vi "PH_Beamline.color PA BL.vi"(0 "i ref in":refnum<vi>, 2 "Color State PA Input":i32, 5 "error in (no error)":errorcluster) -> (14 "i ref out":refnum<vi>, 16 "Color State PA Exit to ED":i32, 17 "Color State PA Exit to MA":i32, 18 "Color State PA Exit to Lab":i32, 19 "error out":errorcluster)   [LabVIEW 2014, in "PH_Beamline.lvlib"]
doc: "This Vi colors the PreAmp beamline elements."
uses:
  PH_Beamline.lvlib
  PH_StatusHandler/PH_StatusHandler.Status.ctl
  PH_Common/PH_Common.lvlib
  PH_BL-Master/PH_BL-Master.lvlib
  PH_StatusHandler/PH_StatusHandler.lvlib
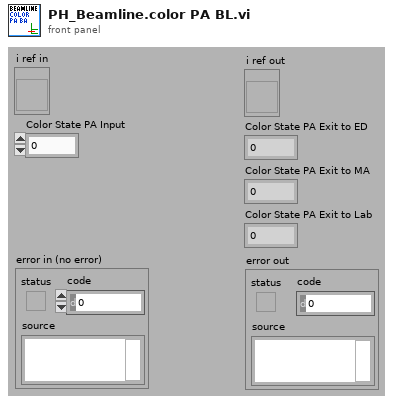
[diagram p1: front panel]
types:
  T1 = typedef "PH_StatusHandler.lvlib/PH_StatusHandler.Status.ctl" = i16
  T2 = typedef "PH_Beamline.lvlib/PH_Beamline.i attribute.ctl" = cluster{"GUI Refs":cluster{"PA ok":refnum<vi>, "MA ok":refnum<vi>, "fs FE ok":refnum<vi>, "ns FE ok":refnum<vi>, "PA ED ok":refnum<vi>, "MAS ok":refnum<vi>, "Booster ok":refnum<vi>, "Mirrortower ok":refnum<vi>, "In.-Box ok":refnum<vi>, "Compressor ok":refnum<vi>, "Experiment LB ok":refnum<vi>, "Experiment LL ok":refnum<vi>, "PHELIX_Beckhoff_Watchdog":refnum<vi>, "Shutters closed":refnum<vi>, "uOPA ok":refnum<vi>, "Vacuum no shotcond Comp LB":refnum<vi>}, "Refs BL MA":refnum<vi>[], "Refs BL MA-IB":refnum<vi>[], "Refs BL fs":refnum<vi>[], "Refs BL PA ED":refnum<vi>[], "Refs BL MAS":refnum<vi>[], "Refs BL Boo":refnum<vi>[], "Refs BL ns":refnum<vi>[], "Refs BL Mirrortower":refnum<vi>[], "Refs BL Compressor":refnum<vi>[], "Refs BL Exp LB":refnum<vi>[], "Radiation Safety":cluster{"Exp Laserbay":cluster{"Ref Op Mode":refnum<vi>, "Ref Laserbay evacuated":refnum<vi>, "Tagname LB evacuated":string, "Shot Mode":T3, "Laserbay evacuated?":i32, "Tagname HV room locked":string, "HV room locked?":i32, "Ref HV room locked":refnum<vi>, "Tagname bridged?":string, "Ref Bridge":refnum<vi>, "I<1E18W/cm²":bool}, "Exp Laserlab":cluster{"Ref Op Mode":refnum<vi>, "Ref Laserlab evacuated":refnum<vi>, "Tagname LL evacuated":string, "Shot Mode":T3, "Laserlab evacuated?":i32, "Tagname bridged?":string, "Ref Bridge":refnum<vi>, "I<1E18W/cm²":bool}}, "Refs BL LL":refnum<vi>[], "PP Igni Heating GUI Refs":refnum<vi>[], "PP Igni Heating Tagnames ":string[], "Refs BL PA":cluster{"undelayed Line before Shutter":refnum<vi>[], "undelayed Line after Shutter":refnum<vi>[], "before Bypass":refnum<vi>[], "delayed Line before Shutter":refnum<vi>[], "delayed Line after Shutter":refnum<vi>[], "before Shutter Input":refnum<vi>[], "after Shutter Input":refnum<vi>[], "Bypass":refnum<vi>[], "before Shutter Exit":refnum<vi>[], "after Shutter Exit":refnum<vi>[], "to MA":refnum<vi>[], "to Lab":refnum<vi>[]}, "BL":cluster{"YLF_BL_Status":i32, "fs_BL_Status":i32, "fs_YLF_BL_Status":i32, "ns_BL_Status":i32, "PA_Input_BL_Status":i32, "PA_UnDelay_BL_Status":i32, "PA_Delay_BL_Status":i32, "PA_BL_Status":i32, "PA_Bypass_BL_Status":i32, "PA_Exit_BL_Status":i32, "PA_LL_BL_Status":i32, "LL_BL_Status":i32, "PA_MA_BL_Status":i32, "MA_Exit_BL_Status":i32, "MA_Z6_BL_Status":i32, "Z6_BL_Status":i32, "MA_LB_BL_Status":i32, "LB_TB2_BL_Status":i32, "PA_before_Bypass_BL_Status":i32, "LB_TB3_BL_Status":i32}, "State Subsystems":cluster{"PA":bool, "MA":bool, "ns FE":bool, "fs FE":bool, "PA ED":bool, "In.-Box":bool, "MAS":bool, "Booster":bool, "Mirrortower":bool, "Compressor":bool, "Experiment LB":bool, "Experiment LL":bool, "uOPA":bool}, "Status Subscriber Information":T4, "Refs BL uOPA":refnum<vi>[], "PA_Input_2_Beam_6PWpGUI not linked?":bool, "PA_Input_Delay_6PGUI not linked?":bool, "Settings":T7}
  T3 = typedef "PH_Beamline.lvlib/PH_Beamline.Operation Mode.ctl" = i32
  T4 = typedef "PH_Beamline.lvlib/PH_Beamline.Status Subscriber Information.ctl" = cluster{"fs Swich YLF":T5, "fs Exit Shutter":T5, "ns Exit Shutter":T5, "PA Input Shutter":T5, "PA PC WP":T5, "PA PC WP 2":T5, "PA Bypass In":T5, "PA Bypass Out":T5, "PA CH 1":T5, "PA delayed":T5, "PA non delayed":T5, "PA Exit Shutter":T5, "PA Switch Lab":T5, "PA Bridge CH Input MA":T5, "MA Diffusor IB":T5, "MA IB Ready":T5, "MA CH 1":T5, "MA CH 2":T5, "MA CH 3":T5, "MA CH 4":T5, "MA Shutter Align Cam":T5, "MA Position MM5":T5, "Calorimeter Switch":T5, "BL Z6 CH 9":T5, "BL Z6 Beamdump":T5, "BL Z6 Shutter":T5, "COS Sensitivity Switch":T5, "Exp LB Shutter":T5, "Exp LB TB 2":T5, "Exp LB TB 3":T5, "PA LL Input CH":T5, "PA LL Output CH":T5, "LL Comp Input Shutter":T5, "LL Comp Output Shutter":T5, "LL Comp FF Shutter":T5, "Exp LL Shutter":T5, "MA IM In IB":T5, "MA IM Out IB":T5, "MA DB In IB":T5, "MA DB Out IB":T5, "Exp LB Shutter Interlock":T5, "Exp LL Shutter Interlock":T5, "MM1 Force Sensor":T5}
  T5 = typedef "PH_BL-Master.lvlib/PH_BL-Master.Status Subscriber Information.ctl" = cluster{"Index of element":i32, "Attributeset":T6}
  T6 = typedef "PH_BL-Master.lvlib/PH_BL-Master.Attribute Set.ctl" = enum16{"Boolean Status Service Subscriber", "Picture Status Service Subscriber"}
  T7 = typedef "PH_Beamline_Chief.lvlib/PH_Beamline_Chief.Settings.ctl" = cluster{"PA Doublepass Mode":bool, "Compressor Vaccuum LB not relevant":bool, "Windowshutter TB2 not relevant":bool, "Windowshutter TB3 not relevant":bool}
  T8 = cluster{"YLF_BL_Status":i32, "fs_BL_Status":i32, "fs_YLF_BL_Status":i32, "ns_BL_Status":i32, "PA_Input_BL_Status":i32, "PA_UnDelay_BL_Status":i32, "PA_Delay_BL_Status":i32, "PA_BL_Status":i32, "PA_Bypass_BL_Status":i32, "PA_Exit_BL_Status":i32, "PA_LL_BL_Status":i32, "LL_BL_Status":i32, "PA_MA_BL_Status":i32, "MA_Exit_BL_Status":i32, "MA_Z6_BL_Status":i32, "Z6_BL_Status":i32, "MA_LB_BL_Status":i32, "LB_TB2_BL_Status":i32, "PA_before_Bypass_BL_Status":i32, "LB_TB3_BL_Status":i32}
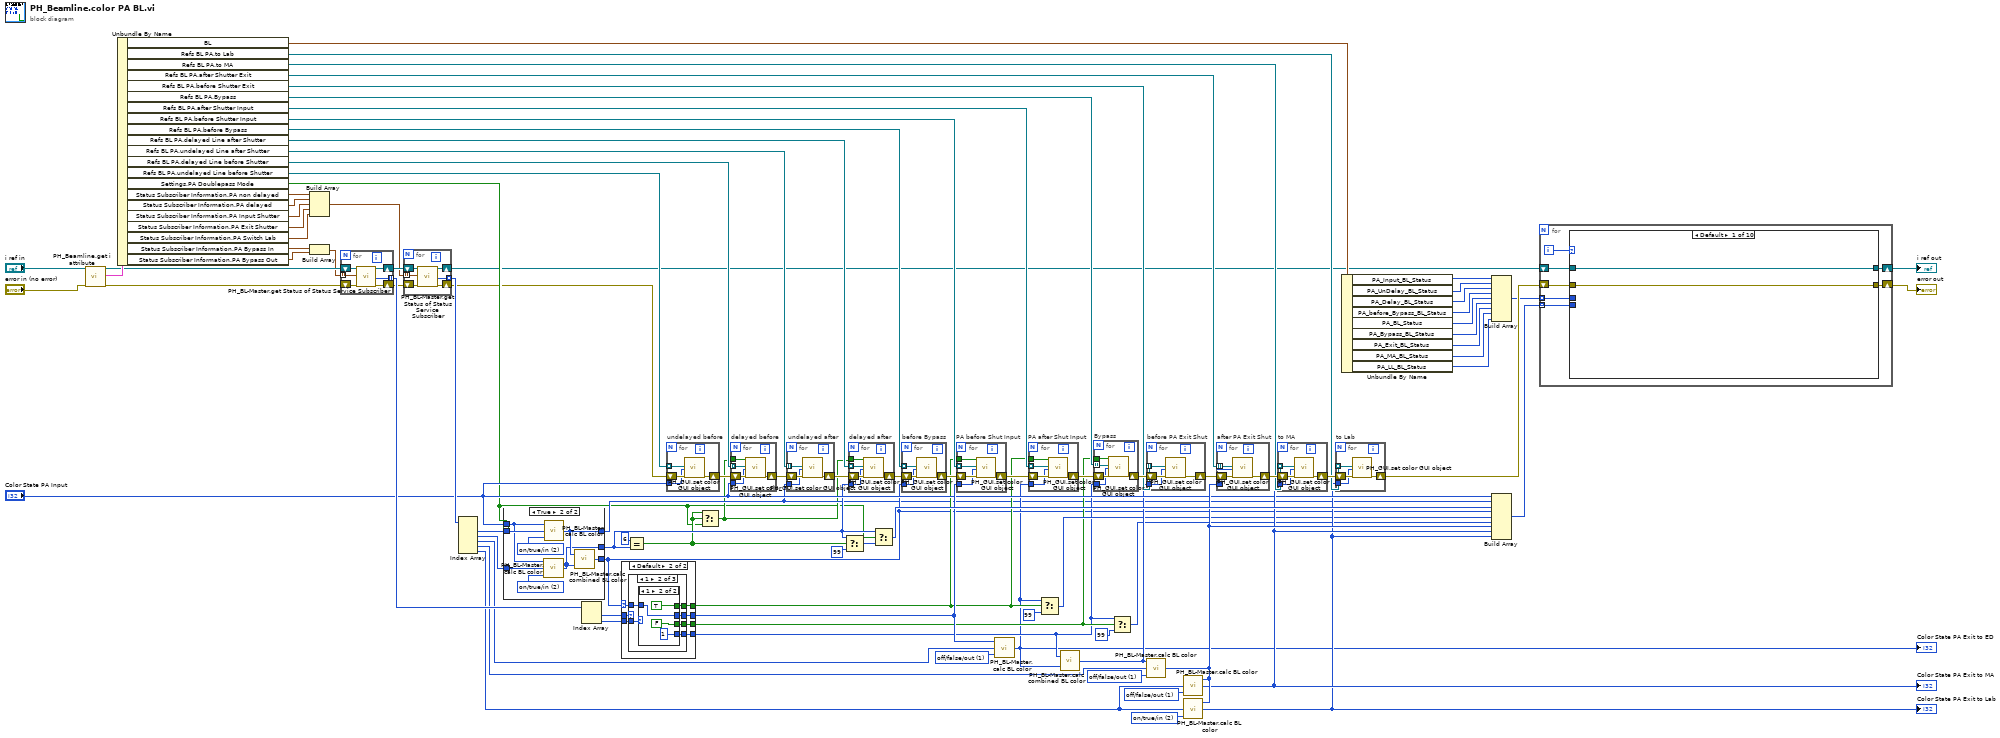
[diagram p0: block diagram]
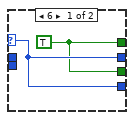
[diagram p2: hidden frame]
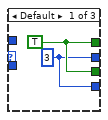
[diagram p3: hidden frame]
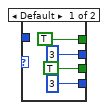
[diagram p4: hidden frame]
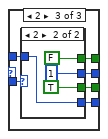
[diagram p5: hidden frame]
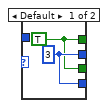
[diagram p6: hidden frame]
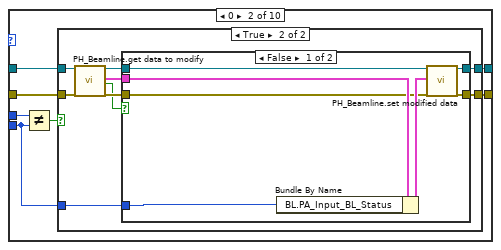
[diagram p8: hidden frame]
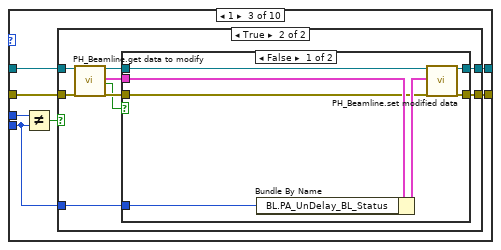
[diagram p11: hidden frame]
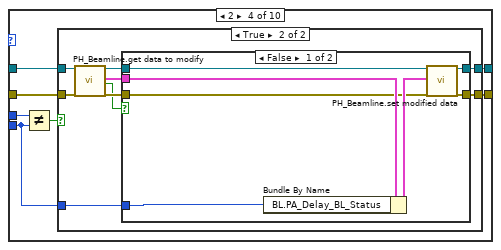
[diagram p14: hidden frame]
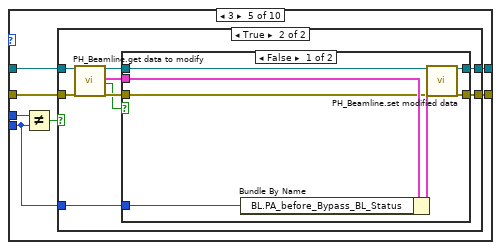
[diagram p17: hidden frame]
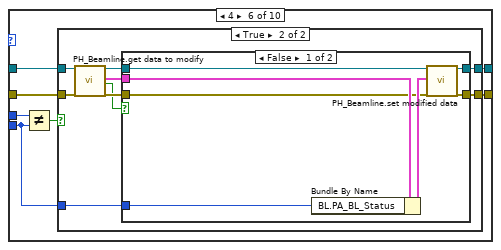
[diagram p20: hidden frame]
diagram:
  w45 = T1 2 items=["no info", "off/false/out", "on/true/in", "Failure", "Alarm", "Status 1", "Status 2", "Status 3"] ("State for \"2\" (on) of ABLE (off/false/out)")
  w46 = T1 1 items=["no info", "off/false/out", "on/true/in", "Failure", "Alarm", "Status 1", "Status 2", "Status 3"] ("State for \"2\" (on) of ABLE (off/false/out)")
  w49 = T1 1 items=["no info", "off/false/out", "on/true/in", "Failure", "Alarm", "Status 1", "Status 2", "Status 3"] ("State for \"2\" (on) of ABLE (off/false/out)")
  w50 = T1 1 items=["no info", "off/false/out", "on/true/in", "Failure", "Alarm", "Status 1", "Status 2", "Status 3"] ("State for \"2\" (on) of ABLE (off/false/out)")
  n1 = call "PH_Beamline.get i attribute.vi"("i ref in"="i ref in", "error in (no error)"="error in (no error)") -> ("i ref out"=w14:refnum<vi>, "i attribute"=w93:T2, "error out"=w13:errorcluster)  [unwired: 15 in]
  n2 = Unbundle By Name(w93) -> ("BL"=w60:T8, "Refs BL PA.to Lab"=w78:refnum<vi>[], "Refs BL PA.to MA"=w77:refnum<vi>[], "Refs BL PA.after Shutter Exit"=w76:refnum<vi>[], "Refs BL PA.before Shutter Exit"=w75:refnum<vi>[], "Refs BL PA.Bypass"=w74:refnum<vi>[], "Refs BL PA.after Shutter Input"=w73:refnum<vi>[], "Refs BL PA.before Shutter Input"=w72:refnum<vi>[], "Refs BL PA.before Bypass"=w42:refnum<vi>[], "Refs BL PA.delayed Line after Shutter"=w71:refnum<vi>[], "Refs BL PA.undelayed Line after Shutter"=w70:refnum<vi>[], "Refs BL PA.delayed Line before Shutter"=w66:refnum<vi>[], "Refs BL PA.undelayed Line before Shutter"=w69:refnum<vi>[], "Settings.PA Doublepass Mode"=w3:bool, "Status Subscriber Information.PA non delayed"=w9:T5, "Status Subscriber Information.PA delayed"=w8:T5, "Status Subscriber Information.PA Input Shutter"=w7:T5, "Status Subscriber Information.PA Exit Shutter"=w6:T5, "Status Subscriber Information.PA Switch Lab"=w5:T5, "Status Subscriber Information.PA Bypass In"=w12:T5, "Status Subscriber Information.PA Bypass Out"=w11:T5)
  n3 = Build Array(w9, w8, w7, w6, w5) -> (w4:T5[])
  n4 = Build Array(w12, w11) -> (w10:T5[])
  n5 = for {
    tunnel: w10 -> [w99] mode=indexing
    shift-right: [w98] -> w88
    shift-left: w14 -> [w97]
    shift-right: [w96] -> w87
    shift-left: w13 -> [w95]
    tunnel: [w94] -> w89 mode=indexing
    n6 = call "PH_BL-Master.get Status of Status Service Subscriber.vi"("i ref in"=w97, "Wanted Status Subscriber Information"=w99, "error in (no error)"=w95) -> ("i ref out"=w98:refnum<vi>, "Status"=w94:T1, "error out"=w96:errorcluster)  [unwired: 11 in, 3 out]
  }
  n7 = for {
    tunnel: [w101] -> w84 mode=indexing
    tunnel: w4 -> [w100] mode=indexing
    shift-right: [w105] -> w2
    shift-left: w87 -> [w102]
    shift-right: [w104] -> w1
    shift-left: w88 -> [w103]
    n8 = call "PH_BL-Master.get Status of Status Service Subscriber.vi"("i ref in"=w103, "Wanted Status Subscriber Information"=w100, "error in (no error)"=w102) -> ("i ref out"=w104:refnum<vi>, "Status"=w101:T1, "error out"=w105:errorcluster)  [unwired: 11 in, 3 out]
  }
  n9 = Index Array(array=w84) -> (element #1=w86:T1, element #2=w85:T1, element #3=w23:T1, element #4=w17:T1, element #5=w24:T1)  [unwired: 5 in]
  n10 = case shown="True" w3 {
    tunnel: "Color State PA Input" -> [w106 w110]
    tunnel: [w106 w109] -> w20
    tunnel: [w106 w108] -> w21
    tunnel: [w106 w107] -> w28
    tunnel: w86 -> [_ w114]
    tunnel: w85 -> [_ w111]
    frame False {
    }
    frame True {
      w112 = T1 2 items=["no info", "off/false/out", "on/true/in", "Failure", "Alarm", "Status 1", "Status 2", "Status 3"] ("State for \"2\" (on) of ABLE (off/false/out)")
      w113 = T1 2 items=["no info", "off/false/out", "on/true/in", "Failure", "Alarm", "Status 1", "Status 2", "Status 3"] ("State for \"2\" (on) of ABLE (off/false/out)")
      n11 = call "PH_BL-Master.calc BL color.vi"("State for \"2\" (on) of ABLE (off/false/out)"=w112, "State ABLE"=w111, "State before ABLE"=w110) -> ("State after ABLE"=w108:i32)
      n12 = call "PH_BL-Master.calc BL color.vi"("State for \"2\" (on) of ABLE (off/false/out)"=w113, "State ABLE"=w114, "State before ABLE"=w110) -> ("State after ABLE"=w109:i32)
      n13 = call "PH_BL-Master.calc combined BL color.vi"("Color State BL 2"=w108, "Color State BL 1"=w109) -> ("Color State combined BL"=w107:i32)
    }
  }
  n14 = Index Array(array=w89) -> (element #1=w83:T1, element #2=w79:T1)  [unwired: 2 in]
  n15 = case shown="Default" w28 {
    selector: w28 -> [w116 w119]
    tunnel: w83 -> [_ w123]
    tunnel: w79 -> [_ w122]
    tunnel: [w116 w121] -> w44
    tunnel: [w116 w120] -> w31
    tunnel: [w115 w118] -> w32
    tunnel: [w115 w117] -> w35
    frame 6 {
      w115 = TRUE
    }
    frame Default {
      n16 = case shown="1" w123 {
        tunnel: [w124 w130 w144] -> w120
        tunnel: [w124 w129 w143] -> w121
        tunnel: w122 -> [_ w131 w145]
        tunnel: w119 -> [_ w128 w142]
        tunnel: [w125 w127 w141] -> w118
        tunnel: [w125 w126 w140] -> w117
        frame Default {
          w125 = TRUE
          w124 = 3
        }
        frame 1 {
          n17 = case shown="1" w131 {
            tunnel: [3 1] -> w130
            tunnel: [3 w137] -> w129
            tunnel: w128 -> [_ w137]
            tunnel: [TRUE FALSE] -> w127
            tunnel: [TRUE TRUE] -> w126
            frame Default {
            }
            frame 1 {
            }
          }
        }
        frame 2 {
          n18 = case shown="2" w145 {
            tunnel: [w147 w150] -> w144
            tunnel: [w147 1] -> w143
            tunnel: w142 -> [_ w150]
            tunnel: [w146 TRUE] -> w141
            tunnel: [w146 FALSE] -> w140
            frame Default {
              w146 = TRUE
              w147 = 3
            }
            frame 2 {
            }
          }
        }
      }
    }
  }
  n19 = Equal?(x=6, y=w21) -> (x = y?=w19:bool)
  n20 = for "undelayed before" {
    tunnel: w69 -> [w155] mode=indexing
    shift-right: [w153] -> w68
    shift-left: w2 -> [w154]
    tunnel: "Color State PA Input" -> [w152]
    n21 = call "PH_GUI.set color GUI object.vi"("GUI object Ref"=w155, "State"=w152, "error in (no error)"=w154) -> ("error out"=w153:errorcluster)  [unwired: 16 in]
  }
  n22 = Select(t=w19, s=w19, f=w3) -> (s? t:f=w18:bool)
  n23 = for "delayed before" {
    tunnel: w66 -> [w160] mode=indexing
    shift-right: [w158] -> w67
    shift-left: w68 -> [w159]
    tunnel: "Color State PA Input" -> [w157]
    tunnel: w18 -> [w156]
    n24 = call "PH_GUI.set color GUI object.vi"("Visible? (true)"=w156, "GUI object Ref"=w160, "State"=w157, "error in (no error)"=w159) -> ("error out"=w158:errorcluster)  [unwired: 15 in]
  }
  n25 = for "undelayed after" {
    tunnel: w70 -> [w164] mode=indexing
    shift-right: [w162] -> w65
    shift-left: w67 -> [w163]
    tunnel: w20 -> [w161]
    n26 = call "PH_GUI.set color GUI object.vi"("GUI object Ref"=w164, "State"=w161, "error in (no error)"=w163) -> ("error out"=w162:errorcluster)  [unwired: 16 in]
  }
  n27 = Select(t=w21, s=w19, f=99) -> (s? t:f=w25:i32)
  n28 = for "delayed after" {
    tunnel: w71 -> [w169] mode=indexing
    shift-right: [w167] -> w64
    shift-left: w65 -> [w168]
    tunnel: w21 -> [w166]
    tunnel: w18 -> [w165]
    n29 = call "PH_GUI.set color GUI object.vi"("Visible? (true)"=w165, "GUI object Ref"=w169, "State"=w166, "error in (no error)"=w168) -> ("error out"=w167:errorcluster)  [unwired: 15 in]
  }
  n30 = Select(t=w21, s=w3, f=w25) -> (s? t:f=w51:i32)
  n31 = for "before Bypass" {
    tunnel: w42 -> [w173] mode=indexing
    shift-right: [w171] -> w41
    shift-left: w64 -> [w172]
    tunnel: w28 -> [w170]
    n32 = call "PH_GUI.set color GUI object.vi"("GUI object Ref"=w173, "State"=w170, "error in (no error)"=w172) -> ("error out"=w171:errorcluster)  [unwired: 16 in]
  }
  n33 = for "PA before Shut Input" {
    tunnel: w72 -> [w178] mode=indexing
    shift-right: [w176] -> w80
    shift-left: w41 -> [w177]
    tunnel: w44 -> [w175]
    tunnel: w35 -> [w174]
    n34 = call "PH_GUI.set color GUI object.vi"("Visible? (true)"=w174, "GUI object Ref"=w178, "State"=w175, "error in (no error)"=w177) -> ("error out"=w176:errorcluster)  [unwired: 15 in]
  }
  n35 = call "PH_BL-Master.calc BL color.vi"("State for \"2\" (on) of ABLE (off/false/out)"=w50, "State ABLE"=w23, "State before ABLE"=w44) -> ("State after ABLE"=w22:i32)
  "Color State PA Exit to ED" <- w22
  n36 = for "PA after Shut Input" {
    tunnel: w73 -> [w183] mode=indexing
    shift-right: [w181] -> w92
    shift-left: w80 -> [w182]
    tunnel: w22 -> [w180]
    tunnel: w35 -> [w179]
    n37 = call "PH_GUI.set color GUI object.vi"("Visible? (true)"=w179, "GUI object Ref"=w183, "State"=w180, "error in (no error)"=w182) -> ("error out"=w181:errorcluster)  [unwired: 15 in]
  }
  n38 = Select(t=w22, s=w35, f=99) -> (s? t:f=w34:i32)
  n39 = call "PH_BL-Master.calc combined BL color.vi"("Color State BL 2"=w22, "Color State BL 1"=w31) -> ("Color State combined BL"=w40:i32)
  n40 = for "Bypass" {
    tunnel: w74 -> [w188] mode=indexing
    shift-right: [w186] -> w91
    shift-left: w92 -> [w187]
    tunnel: w31 -> [w185]
    tunnel: w32 -> [w184]
    n41 = call "PH_GUI.set color GUI object.vi"("Visible? (true)"=w184, "GUI object Ref"=w188, "State"=w185, "error in (no error)"=w187) -> ("error out"=w186:errorcluster)  [unwired: 15 in]
  }
  n42 = Select(t=w31, s=w32, f=99) -> (s? t:f=w30:i32)
  n43 = call "PH_BL-Master.calc BL color.vi"("State for \"2\" (on) of ABLE (off/false/out)"=w49, "State ABLE"=w17, "State before ABLE"=w40) -> ("State after ABLE"=w48:i32)
  n44 = for "before PA Exit Shut" {
    tunnel: w75 -> [w192] mode=indexing
    shift-right: [w190] -> w82
    shift-left: w91 -> [w191]
    tunnel: w40 -> [w189]
    n45 = call "PH_GUI.set color GUI object.vi"("GUI object Ref"=w192, "State"=w189, "error in (no error)"=w191) -> ("error out"=w190:errorcluster)  [unwired: 16 in]
  }
  n46 = call "PH_BL-Master.calc BL color.vi"("State for \"2\" (on) of ABLE (off/false/out)"=w46, "State ABLE"=w24, "State before ABLE"=w48) -> ("State after ABLE"=w47:i32)
  "Color State PA Exit to MA" <- w47
  n47 = call "PH_BL-Master.calc BL color.vi"("State for \"2\" (on) of ABLE (off/false/out)"=w45, "State ABLE"=w24, "State before ABLE"=w48) -> ("State after ABLE"=w37:i32)
  "Color State PA Exit to Lab" <- w37
  n48 = for "after PA Exit Shut" {
    tunnel: w76 -> [w196] mode=indexing
    shift-right: [w194] -> w81
    shift-left: w82 -> [w195]
    tunnel: w48 -> [w193]
    n49 = call "PH_GUI.set color GUI object.vi"("GUI object Ref"=w196, "State"=w193, "error in (no error)"=w195) -> ("error out"=w194:errorcluster)  [unwired: 16 in]
  }
  n50 = for "to MA" {
    tunnel: w77 -> [w200] mode=indexing
    shift-right: [w198] -> w90
    shift-left: w81 -> [w199]
    tunnel: w47 -> [w197]
    n51 = call "PH_GUI.set color GUI object.vi"("GUI object Ref"=w200, "State"=w197, "error in (no error)"=w199) -> ("error out"=w198:errorcluster)  [unwired: 16 in]
  }
  n52 = for "to Lab" {
    tunnel: w78 -> [w204] mode=indexing
    shift-right: [w202] -> w63
    shift-left: w90 -> [w203]
    tunnel: w37 -> [w201]
    n53 = call "PH_GUI.set color GUI object.vi"("GUI object Ref"=w204, "State"=w201, "error in (no error)"=w203) -> ("error out"=w202:errorcluster)  [unwired: 16 in]
  }
  n54 = Unbundle By Name(w60) -> ("PA_Input_BL_Status"=w59:i32, "PA_UnDelay_BL_Status"=w58:i32, "PA_Delay_BL_Status"=w57:i32, "PA_before_Bypass_BL_Status"=w39:i32, "PA_BL_Status"=w56:i32, "PA_Bypass_BL_Status"=w55:i32, "PA_Exit_BL_Status"=w54:i32, "PA_MA_BL_Status"=w53:i32, "PA_LL_BL_Status"=w38:i32)
  n55 = Build Array(w59, w58, w57, w39, w56, w55, w54, w53, w38) -> (w61:i32[])
  n56 = Build Array("Color State PA Input", w20, w51, w28, w34, w30, w48, w47, w37) -> (w52:i32[])
  n57 = for {
    shift-right: [w211] -> w62
    shift-left: w63 -> [w210]
    tunnel: w61 -> [w206] mode=indexing
    tunnel: w52 -> [w207] mode=indexing
    shift-right: [w209] -> w36
    shift-left: w1 -> [w208]
    i -> [w205]
    n58 = case shown="Default" w205 {
      tunnel: [w212 w219 w246 w273 w300 w327 w354 w381 w408 w435] -> w211
      tunnel: w210 -> [w212 w218 w245 w272 w299 w326 w353 w380 w407 w434]
      tunnel: [w213 w217 w244 w271 w298 w325 w352 w379 w406 w433] -> w209
      tunnel: w208 -> [w213 w216 w243 w270 w297 w324 w351 w378 w405 w432]
      tunnel: w207 -> [_ w215 w242 w269 w296 w323 w350 w377 w404 w431]
      tunnel: w206 -> [_ w214 w241 w268 w295 w322 w349 w376 w403 w430]
      frame Default {
      }
      frame 0 {
        n59 = Not Equal?(x=w214, y=w215) -> (x != y?=w220:bool)
        n60 = case shown="True" w220 {
          tunnel: w216 -> [w222 w227]
          tunnel: [w222 w226] -> w217
          tunnel: w218 -> [w221 w225]
          tunnel: [w221 w224] -> w219
          tunnel: w215 -> [_ w223]
          frame False {
          }
          frame True {
            n61 = call "PH_Beamline.get data to modify.vi"("i ref in"=w227, "error in (no error)"=w225) -> ("i ref out"=w230:refnum<vi>, "i attribute"=w228:T2, "timed out"=w229:bool, "error out"=w231:errorcluster)  [unwired: 14 in]
            n62 = case shown="False" w229 {
              tunnel: w231 -> [w232 w239]
              tunnel: w230 -> [w238 w240]
              tunnel: [w237 w239] -> w224
              tunnel: [w236 w240] -> w226
              tunnel: w228 -> [w233 _]
              tunnel: w223 -> [w234 _]
              frame False {
                n63 = Bundle By Name(cluster=w233, "BL.PA_Input_BL_Status"=w234) -> (w235:T2)
                n64 = call "PH_Beamline.set modified data.vi"("i ref in"=w238, "i attribute"=w235, "error in (no error)"=w232) -> ("i ref out"=w236:refnum<vi>, "error out"=w237:errorcluster)  [unwired: 15 in]
              }
              frame True {
              }
            }
          }
        }
      }
      frame 1 {
        n65 = Not Equal?(x=w241, y=w242) -> (x != y?=w247:bool)
        n66 = case shown="True" w247 {
          tunnel: w243 -> [w249 w254]
          tunnel: [w249 w253] -> w244
          tunnel: w245 -> [w248 w252]
          tunnel: [w248 w251] -> w246
          tunnel: w242 -> [_ w250]
          frame False {
          }
          frame True {
            n67 = call "PH_Beamline.get data to modify.vi"("i ref in"=w254, "error in (no error)"=w252) -> ("i ref out"=w257:refnum<vi>, "i attribute"=w255:T2, "timed out"=w256:bool, "error out"=w258:errorcluster)  [unwired: 14 in]
            n68 = case shown="False" w256 {
              tunnel: w258 -> [w259 w266]
              tunnel: w257 -> [w265 w267]
              tunnel: [w264 w266] -> w251
              tunnel: [w263 w267] -> w253
              tunnel: w255 -> [w260 _]
              tunnel: w250 -> [w261 _]
              frame False {
                n69 = Bundle By Name(cluster=w260, "BL.PA_UnDelay_BL_Status"=w261) -> (w262:T2)
                n70 = call "PH_Beamline.set modified data.vi"("i ref in"=w265, "i attribute"=w262, "error in (no error)"=w259) -> ("i ref out"=w263:refnum<vi>, "error out"=w264:errorcluster)  [unwired: 15 in]
              }
              frame True {
              }
            }
          }
        }
      }
      frame 2 {
        n71 = Not Equal?(x=w268, y=w269) -> (x != y?=w274:bool)
        n72 = case shown="True" w274 {
          tunnel: w270 -> [w276 w281]
          tunnel: [w276 w280] -> w271
          tunnel: w272 -> [w275 w279]
          tunnel: [w275 w278] -> w273
          tunnel: w269 -> [_ w277]
          frame False {
          }
          frame True {
            n73 = call "PH_Beamline.get data to modify.vi"("i ref in"=w281, "error in (no error)"=w279) -> ("i ref out"=w284:refnum<vi>, "i attribute"=w282:T2, "timed out"=w283:bool, "error out"=w285:errorcluster)  [unwired: 14 in]
            n74 = case shown="False" w283 {
              tunnel: w285 -> [w286 w293]
              tunnel: w284 -> [w292 w294]
              tunnel: [w291 w293] -> w278
              tunnel: [w290 w294] -> w280
              tunnel: w282 -> [w287 _]
              tunnel: w277 -> [w288 _]
              frame False {
                n75 = Bundle By Name(cluster=w287, "BL.PA_Delay_BL_Status"=w288) -> (w289:T2)
                n76 = call "PH_Beamline.set modified data.vi"("i ref in"=w292, "i attribute"=w289, "error in (no error)"=w286) -> ("i ref out"=w290:refnum<vi>, "error out"=w291:errorcluster)  [unwired: 15 in]
              }
              frame True {
              }
            }
          }
        }
      }
      frame 3 {
        n77 = Not Equal?(x=w295, y=w296) -> (x != y?=w301:bool)
        n78 = case shown="True" w301 {
          tunnel: w297 -> [w303 w308]
          tunnel: [w303 w307] -> w298
          tunnel: w299 -> [w302 w306]
          tunnel: [w302 w305] -> w300
          tunnel: w296 -> [_ w304]
          frame False {
          }
          frame True {
            n79 = call "PH_Beamline.get data to modify.vi"("i ref in"=w308, "error in (no error)"=w306) -> ("i ref out"=w311:refnum<vi>, "i attribute"=w309:T2, "timed out"=w310:bool, "error out"=w312:errorcluster)  [unwired: 14 in]
            n80 = case shown="False" w310 {
              tunnel: w312 -> [w313 w320]
              tunnel: w311 -> [w319 w321]
              tunnel: [w318 w320] -> w305
              tunnel: [w317 w321] -> w307
              tunnel: w309 -> [w314 _]
              tunnel: w304 -> [w315 _]
              frame False {
                n81 = Bundle By Name(cluster=w314, "BL.PA_before_Bypass_BL_Status"=w315) -> (w316:T2)
                n82 = call "PH_Beamline.set modified data.vi"("i ref in"=w319, "i attribute"=w316, "error in (no error)"=w313) -> ("i ref out"=w317:refnum<vi>, "error out"=w318:errorcluster)  [unwired: 15 in]
              }
              frame True {
              }
            }
          }
        }
      }
      frame 4 {
        n83 = Not Equal?(x=w322, y=w323) -> (x != y?=w328:bool)
        n84 = case shown="True" w328 {
          tunnel: w324 -> [w330 w335]
          tunnel: [w330 w334] -> w325
          tunnel: w326 -> [w329 w333]
          tunnel: [w329 w332] -> w327
          tunnel: w323 -> [_ w331]
          frame False {
          }
          frame True {
            n85 = call "PH_Beamline.get data to modify.vi"("i ref in"=w335, "error in (no error)"=w333) -> ("i ref out"=w338:refnum<vi>, "i attribute"=w336:T2, "timed out"=w337:bool, "error out"=w339:errorcluster)  [unwired: 14 in]
            n86 = case shown="False" w337 {
              tunnel: w339 -> [w340 w347]
              tunnel: w338 -> [w346 w348]
              tunnel: [w345 w347] -> w332
              tunnel: [w344 w348] -> w334
              tunnel: w336 -> [w341 _]
              tunnel: w331 -> [w342 _]
              frame False {
                n87 = Bundle By Name(cluster=w341, "BL.PA_BL_Status"=w342) -> (w343:T2)
                n88 = call "PH_Beamline.set modified data.vi"("i ref in"=w346, "i attribute"=w343, "error in (no error)"=w340) -> ("i ref out"=w344:refnum<vi>, "error out"=w345:errorcluster)  [unwired: 15 in]
              }
              frame True {
              }
            }
          }
        }
      }
      frame 5 {
        n89 = Not Equal?(x=w349, y=w350) -> (x != y?=w355:bool)
        n90 = case shown="True" w355 {
          tunnel: w351 -> [w357 w362]
          tunnel: [w357 w361] -> w352
          tunnel: w353 -> [w356 w360]
          tunnel: [w356 w359] -> w354
          tunnel: w350 -> [_ w358]
          frame False {
          }
          frame True {
            n91 = call "PH_Beamline.get data to modify.vi"("i ref in"=w362, "error in (no error)"=w360) -> ("i ref out"=w365:refnum<vi>, "i attribute"=w363:T2, "timed out"=w364:bool, "error out"=w366:errorcluster)  [unwired: 14 in]
            n92 = case shown="False" w364 {
              tunnel: w366 -> [w367 w374]
              tunnel: w365 -> [w373 w375]
              tunnel: [w372 w374] -> w359
              tunnel: [w371 w375] -> w361
              tunnel: w363 -> [w368 _]
              tunnel: w358 -> [w369 _]
              frame False {
                n93 = Bundle By Name(cluster=w368, "BL.PA_Bypass_BL_Status"=w369) -> (w370:T2)
                n94 = call "PH_Beamline.set modified data.vi"("i ref in"=w373, "i attribute"=w370, "error in (no error)"=w367) -> ("i ref out"=w371:refnum<vi>, "error out"=w372:errorcluster)  [unwired: 15 in]
              }
              frame True {
              }
            }
          }
        }
      }
      frame 6 {
        n95 = Not Equal?(x=w376, y=w377) -> (x != y?=w382:bool)
        n96 = case shown="True" w382 {
          tunnel: w378 -> [w384 w389]
          tunnel: [w384 w388] -> w379
          tunnel: w380 -> [w383 w387]
          tunnel: [w383 w386] -> w381
          tunnel: w377 -> [_ w385]
          frame False {
          }
          frame True {
            n97 = call "PH_Beamline.get data to modify.vi"("i ref in"=w389, "error in (no error)"=w387) -> ("i ref out"=w392:refnum<vi>, "i attribute"=w390:T2, "timed out"=w391:bool, "error out"=w393:errorcluster)  [unwired: 14 in]
            n98 = case shown="False" w391 {
              tunnel: w393 -> [w394 w401]
              tunnel: w392 -> [w400 w402]
              tunnel: [w399 w401] -> w386
              tunnel: [w398 w402] -> w388
              tunnel: w390 -> [w395 _]
              tunnel: w385 -> [w396 _]
              frame False {
                n99 = Bundle By Name(cluster=w395, "BL.PA_Exit_BL_Status"=w396) -> (w397:T2)
                n100 = call "PH_Beamline.set modified data.vi"("i ref in"=w400, "i attribute"=w397, "error in (no error)"=w394) -> ("i ref out"=w398:refnum<vi>, "error out"=w399:errorcluster)  [unwired: 15 in]
              }
              frame True {
              }
            }
          }
        }
      }
      frame 7 {
        n101 = Not Equal?(x=w403, y=w404) -> (x != y?=w409:bool)
        n102 = case shown="True" w409 {
          tunnel: w405 -> [w411 w416]
          tunnel: [w411 w415] -> w406
          tunnel: w407 -> [w410 w414]
          tunnel: [w410 w413] -> w408
          tunnel: w404 -> [_ w412]
          frame False {
          }
          frame True {
            n103 = call "PH_Beamline.get data to modify.vi"("i ref in"=w416, "error in (no error)"=w414) -> ("i ref out"=w419:refnum<vi>, "i attribute"=w417:T2, "timed out"=w418:bool, "error out"=w420:errorcluster)  [unwired: 14 in]
            n104 = case shown="False" w418 {
              tunnel: w420 -> [w421 w428]
              tunnel: w419 -> [w427 w429]
              tunnel: [w426 w428] -> w413
              tunnel: [w425 w429] -> w415
              tunnel: w417 -> [w422 _]
              tunnel: w412 -> [w423 _]
              frame False {
                n105 = Bundle By Name(cluster=w422, "BL.PA_MA_BL_Status"=w423) -> (w424:T2)
                n106 = call "PH_Beamline.set modified data.vi"("i ref in"=w427, "i attribute"=w424, "error in (no error)"=w421) -> ("i ref out"=w425:refnum<vi>, "error out"=w426:errorcluster)  [unwired: 15 in]
              }
              frame True {
              }
            }
          }
        }
      }
      frame 8 {
        n107 = Not Equal?(x=w430, y=w431) -> (x != y?=w436:bool)
        n108 = case shown="True" w436 {
          tunnel: w432 -> [w438 w443]
          tunnel: [w438 w442] -> w433
          tunnel: w434 -> [w437 w441]
          tunnel: [w437 w440] -> w435
          tunnel: w431 -> [_ w439]
          frame False {
          }
          frame True {
            n109 = call "PH_Beamline.get data to modify.vi"("i ref in"=w443, "error in (no error)"=w441) -> ("i ref out"=w446:refnum<vi>, "i attribute"=w444:T2, "timed out"=w445:bool, "error out"=w447:errorcluster)  [unwired: 14 in]
            n110 = case shown="False" w445 {
              tunnel: w447 -> [w448 w455]
              tunnel: w446 -> [w454 w456]
              tunnel: [w453 w455] -> w440
              tunnel: [w452 w456] -> w442
              tunnel: w444 -> [w449 _]
              tunnel: w439 -> [w450 _]
              frame False {
                n111 = Bundle By Name(cluster=w449, "BL.PA_LL_BL_Status"=w450) -> (w451:T2)
                n112 = call "PH_Beamline.set modified data.vi"("i ref in"=w454, "i attribute"=w451, "error in (no error)"=w448) -> ("i ref out"=w452:refnum<vi>, "error out"=w453:errorcluster)  [unwired: 15 in]
              }
              frame True {
              }
            }
          }
        }
      }
    }
  }
  "error out" <- w62
  "i ref out" <- w36
